vi "Einheit Index.vi"(8 "Einheit":T1, 11 "Einheit in String":string) -> (3 "Elementindex":i32)   [LabVIEW 2020, in "Linearisierung v2.lvlib" / "SpanEinstellungen.lvlib"]
uses:
  SpanEinstellungen.lvlib
  Einheit.ctl
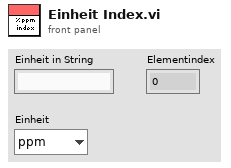
[diagram p1: front panel]
types:
  T1 = typedef "Linearisierung v2.lvlib/SpanEinstellungen.lvlib/Einheit.ctl" = enum16{"ppm", "%"}
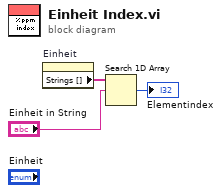
[diagram p0: block diagram]
diagram:
  n1 = property on="Einheit" class="Enum (strikt)"() -> ("Strings []"=w3:string[])  [unwired: 2 in, 2 out]
  n2 = Search 1D Array(1D array=w3, element="Einheit in String") -> (index of element=→"Elementindex":i32)  [unwired: 1 in]
